vi "InstrumentCalibration - Displacement Calibration (SubVI).vi"(8 "error in (no error)":errorcluster, 11 "Motor No":string) -> (0 "error out":errorcluster, 1 "Zero":dbl, 2 "Unit":string, 3 "Displacement":dbl)   [LabVIEW 2019]
uses:
  Controls/FGV States.ctl
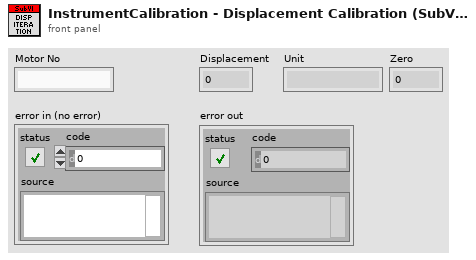
[diagram p1: front panel]
types:
  T1 = typedef "FGV States.ctl" = enum16{"Read", "Write"}
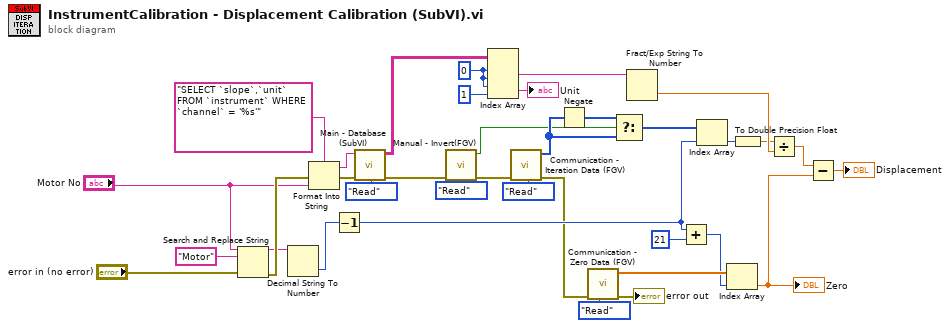
[diagram p0: block diagram]
diagram:
  w14 = 0 ("index (row)")
  n1 = Search and Replace String(input string="Motor No", search string="Motor", error in="error in (no error)") -> (result string=w25:string, error out=w36:errorcluster)  [unwired: 5 in, 2 out]
  n2 = Decimal String To Number(string=w25) -> (number=w26:i32)  [unwired: 2 in, 1 out]
  n3 = Format Into String(format string="SELECT `slope`,`unit` FROM `instrument` WHERE `channel` = '%s'" ("source"), error in=w36, "Motor No") -> (resulting string=w19:string, error out=w20:errorcluster)  [unwired: 1 in]
  n4 = Decrement(x=w26) -> (x-1=w9:i32)
  n5 = call "Main - Database (SubVI).vi"("Enum"=FGV_States."Read", "error in (no error)"=w20, "SQL query"=w19) -> ("error out"=w28:errorcluster, "data"=w21:string[][])  [unwired: 7 in]
  n6 = call "Manual - Invert(FGV).vi"("Action"=FGV_States."Read", "error in (no error)"=w28) -> ("error out"=w29:errorcluster, "invert out"=w31:bool)  [unwired: 8 in]
  n7 = Index Array(array=w21, index (row) #1=w14, index (col) #1=w14, index (row) #2=w14, index (col) #2=1 ("disabled index (col)")) -> (element #1=w22:string, element #2=→"Unit":string)
  n8 = call "Communication - Iteration Data (FGV).vi"("Action"=FGV_States."Read", "error in (no error)"=w29) -> ("error out"=w6:errorcluster, "Iteration SV Out"=w33:i64[])  [unwired: 8 in]
  n9 = Negate(x=w33) -> (-x=w30:i64[])
  n10 = call "Communication - Zero Data (FGV).vi"("Action"=FGV_States."Read", "error in (no error)"=w6) -> ("error out"=→"error out":errorcluster, "Zero Out"=w10:dbl[])  [unwired: 8 in]
  n11 = Select(t=w30, s=w31, f=w33) -> (s? t:f=w32:i64[])
  n12 = Fract/Exp String To Number(string=w22) -> (number=w23:dbl)  [unwired: 3 in, 1 out]
  n13 = Add(x=w9, y=21) -> (x+y=w7:i32)
  n14 = Index Array(array=w32, index=w9) -> (element=w18:i64)
  n15 = Index Array(array=w10, index=w7) -> (element=w4:dbl)
  "Zero" <- w4
  n16 = To Double Precision Float(number=w18) -> (double precision float=w3:dbl)
  n17 = Divide(x=w3, y=w23) -> (x/y=w2:dbl)
  n18 = Subtract(x=w2, y=w4) -> (x-y=→"Displacement":dbl)
